vi "EjemploDragAndDrop.vi"() -> ()   [LabVIEW 2020]
uses:
  <vilib>/measure/NI_MABase.lvlib
panel:
  in  "drop target":dbl[](array[numeric])
  out "drag source":waveform(dbl)(graph)
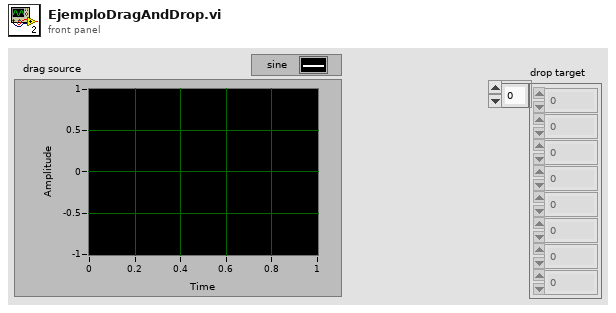
[diagram p1: front panel]
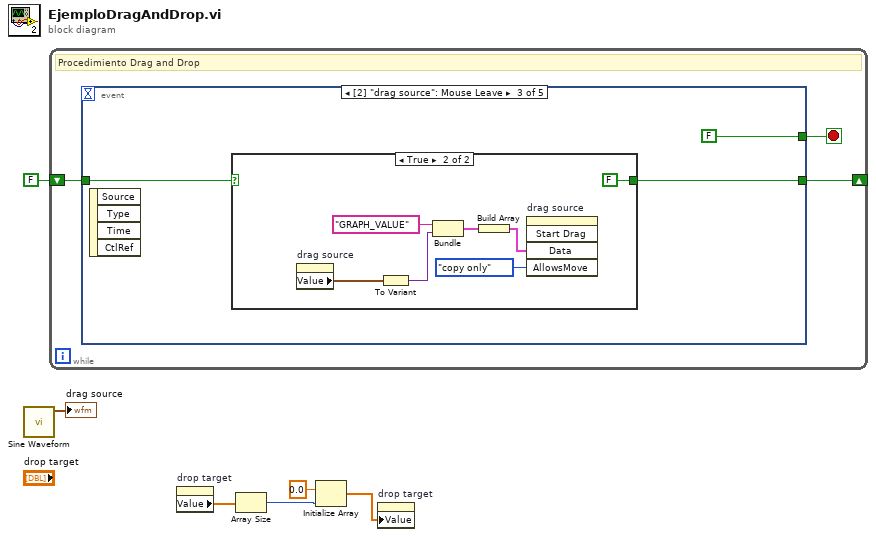
[diagram p0: block diagram]
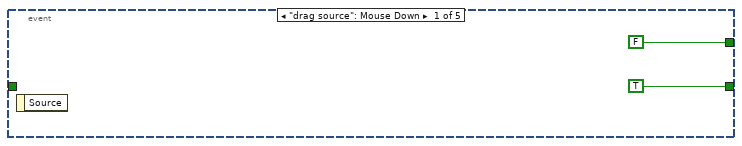
[diagram p2: hidden frame]
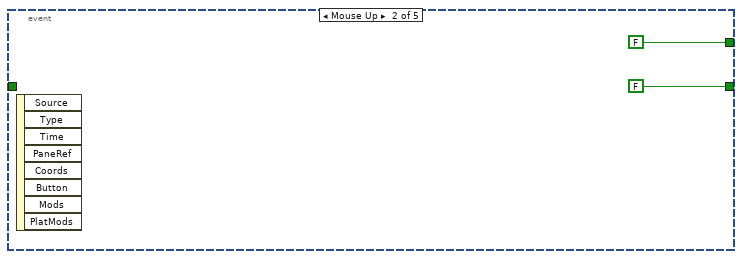
[diagram p3: hidden frame]
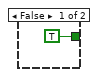
[diagram p4: hidden frame]
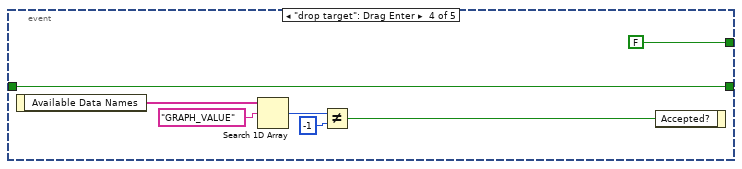
[diagram p5: hidden frame]
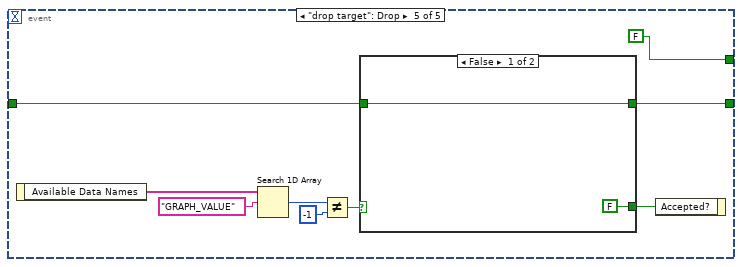
[diagram p6: hidden frame]
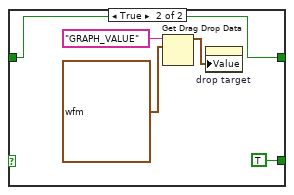
[diagram p7: hidden frame]
diagram:
  n1 = call <vilib>:"Sine Waveform.vi"() -> ("signal out"=→"drag source":waveform(dbl))  [unwired: 10 in, 1 out]
  n2 = while {
    shift-right: [w9] -> _
    shift-left: FALSE -> [w8]
    stop <- w7 stop-if-true
    # "Procedimiento Drag and Drop"
    n3 = event shown="[2] \"drag source\": Mouse Leave" {
      selector: _ -> [_ _ _ _ _]
      dyn-events: _ -> [_ _ _ _ _]
      timeout: _ -> [_ _ _ _ _]
      tunnel: [TRUE FALSE w15 w30 w34] -> w9
      tunnel: w8 -> [_ _ w16 w30 w35]
      tunnel: [FALSE FALSE FALSE FALSE FALSE] -> w7
      event "drag source": Mouse Down {
        n4 = event-data() -> ()  [unwired: 1 in, 1 out]
      }
      event Mouse Up {
        n5 = event-data() -> ()  [unwired: 1 in, 8 out]
      }
      event "drag source": Mouse Leave {
        n6 = event-data() -> ()  [unwired: 1 in, 4 out]
        n7 = case shown="True" w16 {
          tunnel: [TRUE FALSE] -> w15
          frame False {
          }
          frame True {
            n8 = property on="drag source" class="WFGraph (strict)"() -> ("Value"=w23:waveform(dbl))  [unwired: 2 in, 2 out]
            n9 = To Variant(anything=w23) -> (Variant=w21:variant)
            n10 = Bundle("GRAPH_VALUE", "Variant"=w21) -> (w20:cluster{string, "Variant":variant})  [unwired: 1 in]
            n11 = Build Array(w20) -> (w19:cluster{string, "Variant":variant}[])
            n12 = invoke on="drag source" class="WFGraph (strict)" method="Start Drag"("Data"=w19, "AllowsMove"=enum32{"copy or move", "copy only", "move only"}."copy only" ("Drag Mode")) -> ()  [unwired: 3 in, 5 out]
          }
        }
      }
      event "drop target": Drag Enter {
        n13 = event-data() -> ("Available Data Names"=w29:string[])  [unwired: 1 in]
        n14 = Search 1D Array(1D array=w29, element="GRAPH_VALUE") -> (index of element=w27:i32)  [unwired: 1 in]
        n15 = Not Equal?(x=w27, y=-1) -> (x != y?=w25:bool)
        n16 = event-data("Accepted?"=w25) -> ()  [unwired: 1 in, 1 out]
      }
      event "drop target": Drop {
        n17 = event-data() -> ("Available Data Names"=w40:string[])  [unwired: 1 in]
        n18 = Search 1D Array(1D array=w40, element="GRAPH_VALUE") -> (index of element=w37:i32)  [unwired: 1 in]
        n19 = Not Equal?(x=w37, y=-1) -> (x != y?=w32:bool)
        n20 = case shown="False" w32 {
          tunnel: w35 -> [w41 w44]
          tunnel: [w41 w44] -> w34
          tunnel: [FALSE TRUE] -> w33
          frame False {
          }
          frame True {
            n21 = Get Drag Drop Data(8:waveform(dbl) {"t0"=timestamp(0 s since 1904-01-01), "dt"=1.0, "Y"=[]} ("drag source"), 9:"GRAPH_VALUE" ("element")) -> (3:w45:waveform(dbl))  [unwired: 1 in, 1 out]
            n22 = property on="drop target" class="Arr (strict)"("Value"=w45) -> ()  [unwired: 2 in, 2 out]
          }
        }
        n23 = event-data("Accepted?"=w33) -> ()  [unwired: 1 in, 1 out]
      }
    }
  }
  n24 = property on="drop target" class="Arr (strict)"() -> ("Value"=w4:dbl[])  [unwired: 2 in, 2 out]
  n25 = Array Size(array=w4) -> (size(s)=w3:i32)
  n26 = Initialize Array(0.0 ("element"), w3) -> (w1:dbl[])
  n27 = property on="drop target" class="Arr (strict)"("Value"=w1) -> ()  [unwired: 2 in, 2 out]
